vi "Create DOs.vi"(0 "reference in":refnum<class "Stand.lvclass">, 11 "error in (no error)":errorcluster) -> (4 "reference out":refnum<class "Stand.lvclass">, 15 "error out":errorcluster)   [LabVIEW 2019, in "Stand.lvclass"]
uses:
  Stand.lvclass
  C:/Users/ANENKOV_V1/Desktop/src/Proccess_class/Proccess.lvclass
  Stand.lvclass/Stand.ctl
  Proccess_class/Proccess.lvclass/Proccess.ctl
  Proccess_class/TAGs.ctl
  DO_class/DO.lvclass
  Proccess_class/Proccess.lvclass
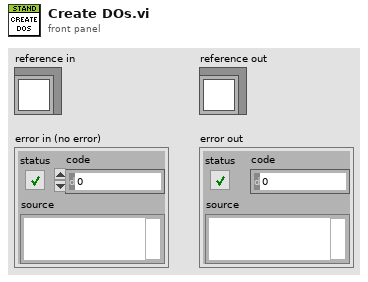
[diagram p1: front panel]
types:
  T1 = typedef "Proccess.lvclass/TAGs.ctl" = cluster{"TAG":string, "PTAG":string, "DESC":string}
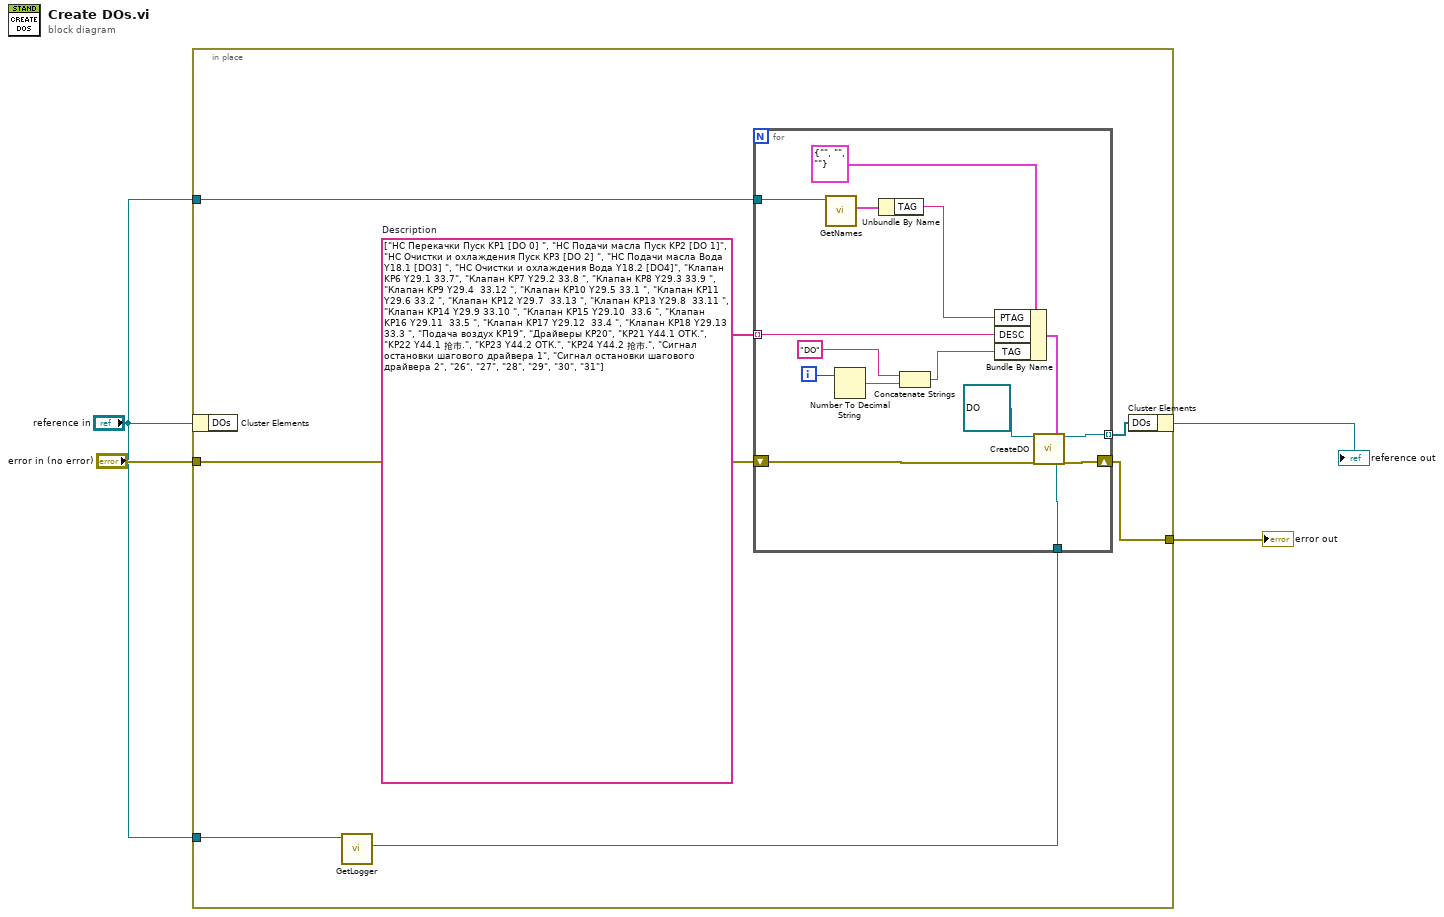
[diagram p0: block diagram]
diagram:
  n1 = in-place {
    in-place-border: "error in (no error)" -> [w11]
    in-place-border: "reference in" -> [w9]
    in-place-border: "reference in" -> [w8]
    in-place-border: [w5] -> w4
    w6 = string[] ["НС Перекачки Пуск KP1 [DO 0] ", "НС Подачи масла Пуск KP2 [DO 1]", "НС Очистки и охлаждения Пуск KP3 [DO 2] ", "НС Подачи масла Вода Y18.1 [DO3] ", "НС Очистки и охлаждения Вода Y18.2 [DO4]", "Клапан KP6 Y29.1 33.7", "Клапан KP7 Y29.2 33.8 ", "Клапан KP8 Y29.3 33.9 ", "Клапан KP9 Y29.4  33.12 ", "Клапан KP10 Y29.5 33.1 ", "Клапан KP11 Y29.6 33.2 ", "Клапан KP12 Y29.7  33.13 ", "Клапан KP13 Y29.8  33.11 ", "Клапан KP14 Y29.9 33.10 ", "Клапан KP15 Y29.10  33.6 ", "Клапан KP16 Y29.11  33.5 ", "Клапан KP17 Y29.12  33.4 ", "Клапан KP18 Y29.13 33.3 ", "Подача воздух KP19", "Драйверы KP20", "KP21 Y44.1 ОТК.", "KP22 Y44.1 抢市.", "KP23 Y44.2 ОТК.", "KP24 Y44.2 抢市.", "Сигнал остановки шагового драйвера 1", "Сигнал остановки шагового драйвера 2", "26", "27", "28", "29", "30", "31"]  # Description
    n2 = in-place-cluster #1("reference in") -> ()  [unwired: 1 out]
    n3 = call "GetLogger.vi"("Proccess in"=w8) -> ("Logger"=w7:refnum<class "Logger.lvclass">)  [unwired: 10 in]
    n4 = for {
      tunnel: [w22] -> w10 mode=indexing
      shift-right: [w21] -> w5
      shift-left: w11 -> [w23]
      tunnel: w6 -> [w17] mode=indexing
      tunnel: w9 -> [w14]
      tunnel: w7 -> [w13]
      i -> [w26]
      n5 = call "GetNames.vi"("Proccess in"=w14) -> ("Tags"=w16:T1)  [unwired: 10 in]
      n6 = Number To Decimal String(number=w26) -> (decimal integer string=w25:string)  [unwired: 1 in]
      n7 = Unbundle By Name(w16) -> ("TAG"=w15:string)
      n8 = Concatenate Strings("DO" ("string"), w25) -> (w18:string)
      n9 = Bundle By Name(cluster=T1 {"TAG"="", "PTAG"="", "DESC"=""} ("Tags"), "PTAG"=w15, "DESC"=w17, "TAG"=w18) -> (w19:T1)
      n10 = call "CreateDO.vi"("Sig_DI_Simple in"=refnum<class "DO.lvclass"> refnum, "error in (no error)"=w23, "Tags"=w19, "Logger"=w13) -> ("Sig_DI_Simple out"=w22:refnum<class "DO.lvclass">, "error out"=w21:errorcluster)  [unwired: 14 in]
    }
    n11 = in-place-cluster #1("DOs"=w10) -> (→"reference out":refnum<class "Stand.lvclass">)
  }
  "error out" <- w4
